vi "Request Daemon Termination.vi"(8 "error in (no error)":errorcluster, 10 "element":T1={"Termination Reason"=enum."Goodbye Received", "Error URI"="wamp.error.protocol_violation", "Message"="", "Terminate?"=FALSE}, 11 "queue":refnum<queue>) -> (0 "error out":errorcluster)   [LabVIEW 2020, in "wamplv.lvlib" / "WAMP Client.lvclass"]
uses:
  <userlib>/wamplv/WAMP Client/WAMP Client.lvclass
  <userlib>/wamplv/WAMP Client/TypeDef/Daemon Termination Request.ctl
  <userlib>/wamplv/WAMP Client/TypeDef/Daemon Termination Reason.ctl
  <userlib>/wamplv/WAMP Client/WAMP Client.lvclass/WAMP Client.ctl
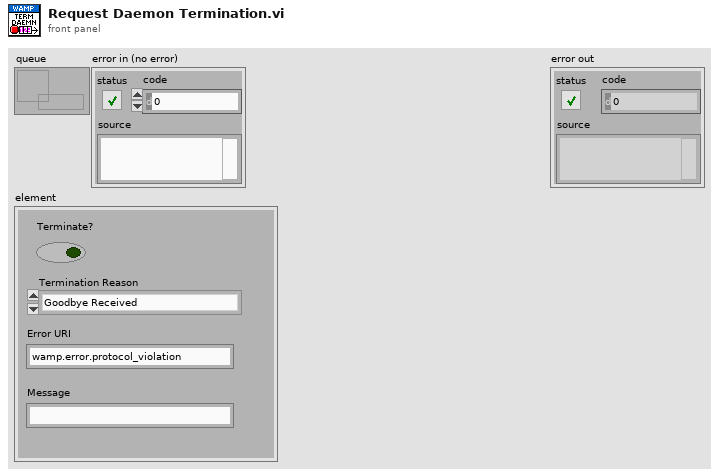
[diagram p1: front panel]
types:
  T1 = typedef "wamplv.lvlib/WAMP Client.lvclass/Daemon Termination Request.ctl" = cluster{"Termination Reason":T2, "Error URI":string, "Message":string, "Terminate?":bool}
  T2 = typedef "wamplv.lvlib/WAMP Client.lvclass/Daemon Termination Reason.ctl" = enum16{"Goodbye Received", "Abort Received", "Send Goodbye", "Send Abort", "Read Loop Failure", "Write Loop Failure", "Message Loop Failure"}
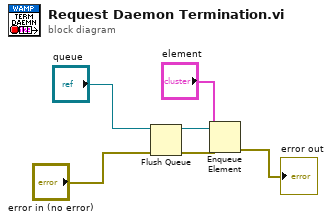
[diagram p0: block diagram]
diagram:
  n1 = Flush Queue(queue="queue", error in (no error)="error in (no error)") -> (queue out=w6:refnum<queue>, error out=w5:errorcluster)  [unwired: 1 out]
  n2 = Enqueue Element(queue=w6, element="element", error in (no error)=w5) -> (error out=→"error out":errorcluster)  [unwired: 1 in, 2 out]
